vi "KB-DealWith All Picture.vi"(0 "ImageArray":T1[](array[typedef]), 5 "Param List CCD":string[][](array[string])=[[";1650.000;1055.000;162.000;324.000;0.000;0.000;0;1;3;3;15.000;4;0;1;0;0;1;65280;255;16776960;16711680;", ";1645.000;1058.000;62.000;156.000;0.000;0.000;0;1;13;13;52.000;4;0;1;0;0;1;65280;255;16776960;16711680;", "Null", "Null", "Null", "Null", "Null", "Null", "Null", "Null"], [";1666.000;992.000;164.000;329.000;0.000;0.000;0;1;3;3;12.000;4;0;1;0;0;1;65280;255;16776960;16711680;", ";1644.000;989.000;75.000;150.000;0.000;0.000;0;2;13;13;52.000;4;0;1;0;0;1;65280;255;16776960;16711680;", "Null", "Null", "Null", "Null", "Null", "Null", "Null", "Null"], [";1641.000;1097.000;175.000;301.000;0.000;0.000;0;1;3;3;12.000;4;0;1;0;0;1;65280;255;16776960;16711680;", ";1637.000;1088.000;74.000;149.000;0.000;0.000;0;2;13;13;52.000;4;0;1;0;0;1;65280;255;16776960;16711680;", "Null", "Null", "Null", "Null", "Null", "Null", "Null", "Null"], [";1645.000;1085.000;198.000;330.000;0.000;0.000;0;1;3;3;12.000;4;0;1;0;0;1;65280;255;16776960;16711680;", ";1649.000;1092.000;69.000;146.000;0.000;0.000;0;2;13;13;52.000;4;0;1;0;0;1;65280;255;16776960;16711680;", "Null", "Null", "Null", "Null", "Null", "Null", "Null", "Null"], [";1646.000;1097.000;198.000;323.000;0.000;0.000;0;1;3;3;12.000;4;0;1;0;0;1;65280;255;16776960;16711680;", ";1647.000;1093.000;74.000;149.000;0.000;0.000;0;2;19;13;52.000;4;0;1;0;0;1;65280;255;16776960;16711680;", "Null", "Null", "Null", "Null", "Null", "Null", "Null", "Null"], [";1650.000;1035.000;192.000;317.000;0.000;0.000;0;1;3;3;12.000;4;0;1;0;0;1;65280;255;16776960;16711680;", ";1669.000;1059.000;33.000;161.000;0.000;0.000;0;2;19;13;52.000;4;0;1;0;0;1;65280;255;16776960;16711680;", "Null", "Null", "Null", "Null", "Null", "Null", "Null", "Null"], [";1549.000;1024.000;204.000;306.000;0.000;0.000;0;1;3;3;12.000;4;0;1;0;0;1;65280;255;16776960;16711680;", ";1546.000;1027.000;72.000;144.000;0.000;0.000;0;2;19;13;52.000;4;0;1;0;0;1;65280;255;16776960;16711680;", "Null", "Null", "Null", "Null", "Null", "Null", "Null", "Null"], [";1552.000;926.000;174.000;303.000;0.000;0.000;0;1;19;13;52.000;4;0;1;0;0;1;65280;255;16776960;16711680;", ";1553.000;934.000;72.000;145.000;0.000;0.000;0;2;19;13;52.000;4;0;1;0;0;1;65280;255;16776960;16711680;", "Null", "Null", "Null", "Null", "Null", "Null", "Null", "Null"], [";1546.000;954.000;166.000;315.000;0.000;0.000;0;1;3;3;12.000;4;0;1;0;0;1;65280;255;16776960;16711680;", ";1547.000;950.000;73.000;147.000;0.000;0.000;0;2;19;13;52.000;4;0;1;0;0;1;65280;255;16776960;16711680;", "Null", "Null", "Null", "Null", "Null", "Null", "Null", "Null"], [";1543.000;971.000;184.000;314.000;0.000;0.000;0;1;3;3;12.000;4;0;1;0;0;1;65280;255;16776960;16711680;", ";1547.000;972.000;76.000;152.000;0.000;0.000;0;2;19;13;52.000;4;0;1;0;0;1;65280;255;16776960;16711680;", "Null", "Null", "Null", "Null", "Null", "Null", "Null", "Null"], [";1552.000;1013.000;185.000;317.000;0.000;0.000;0;1;3;3;12.000;4;0;1;0;0;1;65280;255;16776960;16711680;", ";1549.000;1013.000;72.000;145.000;0.000;0.000;0;2;19;13;52.000;4;0;1;0;0;1;65280;255;16776960;16711680;", "Null", "Null", "Null", "Null", "Null", "Null", "Null", "Null"], [";1560.000;910.000;181.000;316.000;0.000;0.000;0;1;3;3;12.000;4;0;1;0;0;1;65280;255;16776960;16711680;", ";1562.000;918.000;70.000;140.000;0.000;0.000;0;1;19;13;52.000;4;0;1;0;0;1;65280;255;16776960;16711680;", "Null", "Null", "Null", "Null", "Null", "Null", "Null", "Null"], [";1330.000;923.000;139.000;279.000;0.000;0.000;0;2;21;13;15.000;4;0;1;0;0;1;65280;255;16776960;16711680;", ";1328.000;918.000;70.000;141.000;0.000;0.000;0;2;21;13;45.000;4;0;1;0;0;1;65280;255;16776960;16711680;", "Null", "Null", "Null", "Null", "Null", "Null", "Null", "Null"], [";1370.000;1170.000;162.000;278.000;0.000;0.000;0;2;21;13;15.000;4;0;1;0;0;1;65280;255;16776960;16711680;", ";1367.000;1164.000;71.000;143.000;0.000;0.000;0;2;19;13;15.000;4;0;1;0;0;1;65280;255;16776960;16711680;", "Null", "Null", "Null", "Null", "Null", "Null", "Null", "Null"], [";1660.000;1110.000;150.000;301.000;0.000;0.000;0;2;21;13;15.000;4;0;1;0;0;1;65280;255;16776960;16711680;", ";1662.000;1114.000;78.000;156.000;0.000;0.000;0;2;21;13;25.000;4;0;1;0;0;1;65280;255;16776960;16711680;", "Null", "Null", "Null", "Null", "Null", "Null", "Null", "Null"], [";1611.000;1132.000;156.000;273.000;0.000;0.000;0;2;21;13;45.000;4;0;1;0;0;1;65280;255;16776960;16711680;", ";1613.000;1132.000;72.000;145.000;0.000;0.000;0;2;21;13;15.000;4;0;1;0;0;1;65280;255;16776960;16711680;", "Null", "Null", "Null", "Null", "Null", "Null", "Null", "Null"], [";1591.000;1169.000;165.000;294.000;0.000;0.000;0;1;13;13;15.000;4;0;1;0;0;1;65280;255;16776960;16711680;", ";1625.000;1187.000;75.000;150.000;0.000;0.000;0;2;13;13;55.000;4;0;1;0;0;1;65280;255;16776960;16711680;", "Null", "Null", "Null", "Null", "Null", "Null", "Null", "Null"], [";1586.000;1193.000;179.000;359.000;0.000;0.000;0;1;13;13;35.000;4;0;1;0;0;1;65280;255;16776960;16711680;", ";1614.000;1212.000;75.000;150.000;0.000;0.000;0;2;13;13;55.000;4;0;1;0;0;1;65280;255;16776960;16711680;", "Null", "Null", "Null", "Null", "Null", "Null", "Null", "Null"], [";1676.000;1155.000;175.000;350.000;0.000;0.000;0;1;13;13;55.000;4;0;1;0;0;1;65280;255;16776960;16711680;", ";1670.000;1157.000;70.000;141.000;0.000;0.000;0;2;13;13;55.000;4;0;1;0;0;1;65280;255;16776960;16711680;", "Null", "Null", "Null", "Null", "Null", "Null", "Null", "Null"], [";1620.000;1151.000;188.000;377.000;0.000;0.000;0;1;13;13;55.000;4;0;1;0;0;1;65280;255;16776960;16711680;", ";1613.000;1143.000;81.000;150.000;0.000;0.000;0;2;13;13;55.000;4;0;1;0;0;1;65280;255;16776960;16711680;", "Null", "Null", "Null", "Null", "Null", "Null", "Null", "Null"], [";1592.000;1152.000;179.000;359.000;0.000;0.000;0;1;13;13;55.000;4;0;1;0;0;1;65280;255;16776960;16711680;", ";1577.000;1142.000;75.000;151.000;0.000;0.000;0;2;13;13;55.000;4;0;1;0;0;1;65280;255;16776960;16711680;", "Null", "Null", "Null", "Null", "Null", "Null", "Null", "Null"], [";1284.000;1016.000;459.000;919.000;0.000;0.000;0;1;13;13;15.000;4;0;1;0;0;1;65280;255;16776960;16711680;", ";1286.000;1055.000;239.000;466.000;0.000;0.000;0;2;13;13;55.000;4;0;1;0;0;1;65280;255;16776960;16711680;", "Null", "Null", "Null", "Null", "Null", "Null", "Null", "Null"], [";1600.000;1172.000;534.000;991.000;0.000;0.000;0;1;13;13;15.000;4;0;1;0;0;1;65280;255;16776960;16711680;", ";1604.000;1188.000;203.000;406.000;0.000;0.000;0;2;15;13;43.000;4;0;1;0;0;1;65280;255;16776960;16711680;", "Null", "Null", "Null", "Null", "Null", "Null", "Null", "Null"], [";1836.000;828.000;597.000;1195.000;0.000;0.000;0;1;15;13;13.000;4;0;1;0;0;1;65280;255;16776960;16711680;", ";1840.000;824.000;216.000;432.000;0.000;0.000;0;2;5;13;43.000;4;0;1;0;0;1;65280;255;16776960;16711680;", "Null", "Null", "Null", "Null", "Null", "Null", "Null", "Null"], [";1583.000;947.000;487.000;975.000;0.000;0.000;0;1;13;13;13.000;4;0;1;0;0;1;65280;255;16776960;16711680;", ";1583.000;941.000;211.000;397.000;0.000;0.000;0;2;5;13;43.000;4;0;1;0;0;1;65280;255;16776960;16711680;", "Null", "Null", "Null", "Null", "Null", "Null", "Null", "Null"], [";1841.000;926.000;497.000;995.000;0.000;0.000;0;1;13;13;13.000;4;0;1;0;0;1;65280;255;16776960;16711680;", ";1820.000;924.000;209.000;418.000;0.000;0.000;0;2;13;13;13.000;4;0;1;0;0;1;65280;255;16776960;16711680;", "Null", "Null", "Null", "Null", "Null", "Null", "Null", "Null"], [";1728.000;864.000;582.000;1165.000;0.000;0.000;0;1;13;13;13.000;4;0;1;0;0;1;65280;255;16776960;16711680;", ";1720.000;888.000;203.000;406.000;0.000;0.000;0;2;13;13;13.000;4;0;1;0;0;1;65280;255;16776960;16711680;", "Null", "Null", "Null", "Null", "Null", "Null", "Null", "Null"], [";1508.000;1012.000;497.000;878.000;0.000;0.000;0;1;13;13;13.000;4;0;1;0;0;1;65280;255;16776960;16711680;", ";1520.000;1008.000;206.000;413.000;0.000;0.000;0;2;13;13;13.000;4;0;1;0;0;1;65280;255;16776960;16711680;", "Null", "Null", "Null", "Null", "Null", "Null", "Null", "Null"], [";2110.000;860.000;450.000;901.000;0.000;0.000;0;1;13;13;13.000;4;0;1;0;0;1;65280;255;16776960;16711680;", ";2105.000;860.000;205.000;410.000;0.000;0.000;0;2;15;13;13.000;4;0;1;0;0;1;65280;255;16776960;16711680;", "Null", "Null", "Null", "Null", "Null", "Null", "Null", "Null"], [";1900.000;1200.000;491.000;983.000;0.000;0.000;0;1;15;13;13.000;4;0;1;0;0;1;65280;255;16776960;16711680;", ";1877.000;1223.000;205.000;411.000;0.000;0.000;0;2;19;13;55.000;4;0;1;0;0;1;65280;255;16776960;16711680;", "Null", "Null", "Null", "Null", "Null", "Null", "Null", "Null"], [";2850.000;740.000;530.000;933.000;0.000;0.000;0;1;13;13;15.000;4;0;1;0;0;1;65280;255;16776960;16711680;", ";2849.000;737.000;215.000;404.000;0.000;0.000;0;2;13;13;15.000;4;0;1;0;0;1;65280;255;16776960;16711680;", "Null", "Null", "Null", "Null", "Null", "Null", "Null", "Null"], ["Null", "Null", "Null", "Null", "Null", "Null", "Null", "Null", "Null", "Null"], ["Null", "Null", "Null", "Null", "Null", "Null", "Null", "Null", "Null", "Null"]], 7 "Radio Array":string[](array[string])=["0.0079533404029692", "0.0065116279069767"], 9 "平面":i32=3000, 11 "侧面":i32=43000) -> (4 "Left Data":string[][](array[string]))   [LabVIEW 2015]
uses:
  <vilib>/vision/Image Controls.llb/IMAQ Image.ctl
panel:
  out "x/y":dbl
  out "毫秒计时值":u32
  out "路径":path
  out "数值":i32
  out "Item31":string[](array[string])
  out "Item30":string[](array[string])
  out "Item29":string[](array[string])
  out "Item28":string[](array[string])
  out "Item27":string[](array[string])
  out "Item26":string[](array[string])
  out "Item25":string[](array[string])
  out "Item24":string[](array[string])
  out "Item23":string[](array[string])
  out "Item22":string[](array[string])
  out "Item21":string[](array[string])
  out "Item20":string[](array[string])
  out "Item19":string[](array[string])
  out "Item18":string[](array[string])
  out "Item17":string[](array[string])
  out "Item16":string[](array[string])
  out "Item15":string[](array[string])
  out "Item14":string[](array[string])
  out "Item13":string[](array[string])
  out "Item12":string[](array[string])
  out "Item11":string[](array[string])
  out "Item10":string[](array[string])
  out "Item9":string[](array[string])
  out "Item8":string[](array[string])
  out "Item7":string[](array[string])
  out "Item6":string[](array[string])
  out "Item5":string[](array[string])
  out "Item4":string[](array[string])
  out "Item3":string[](array[string])
  out "Item2":string[](array[string])
  out "Item1":string[](array[string])
  out "CCD 2":string
  out "CCD 1":string
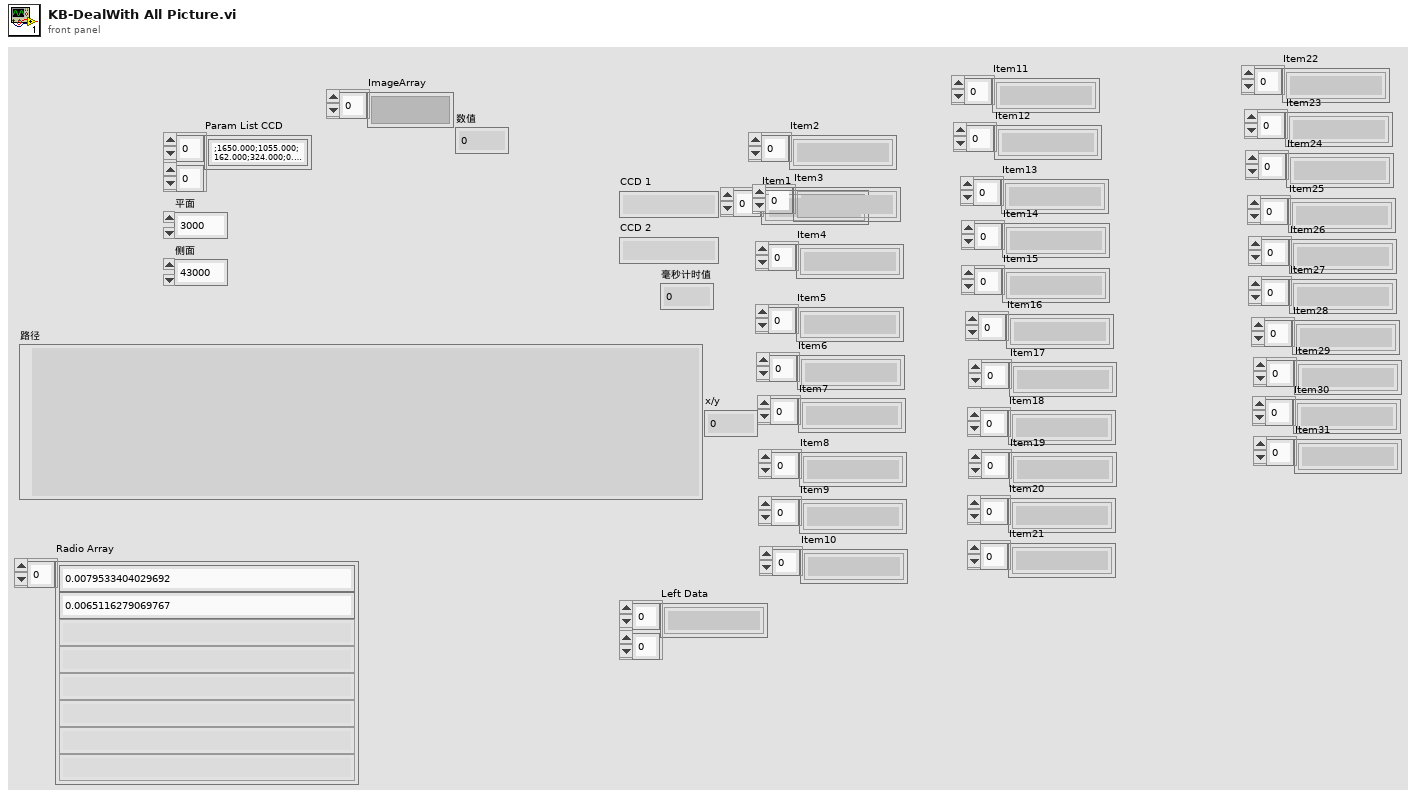
[diagram p1: front panel]
types:
  T1 = typedef "IMAQ Image.ctl" = refnum<image>
  T2 = typedef "Image Type" = u32
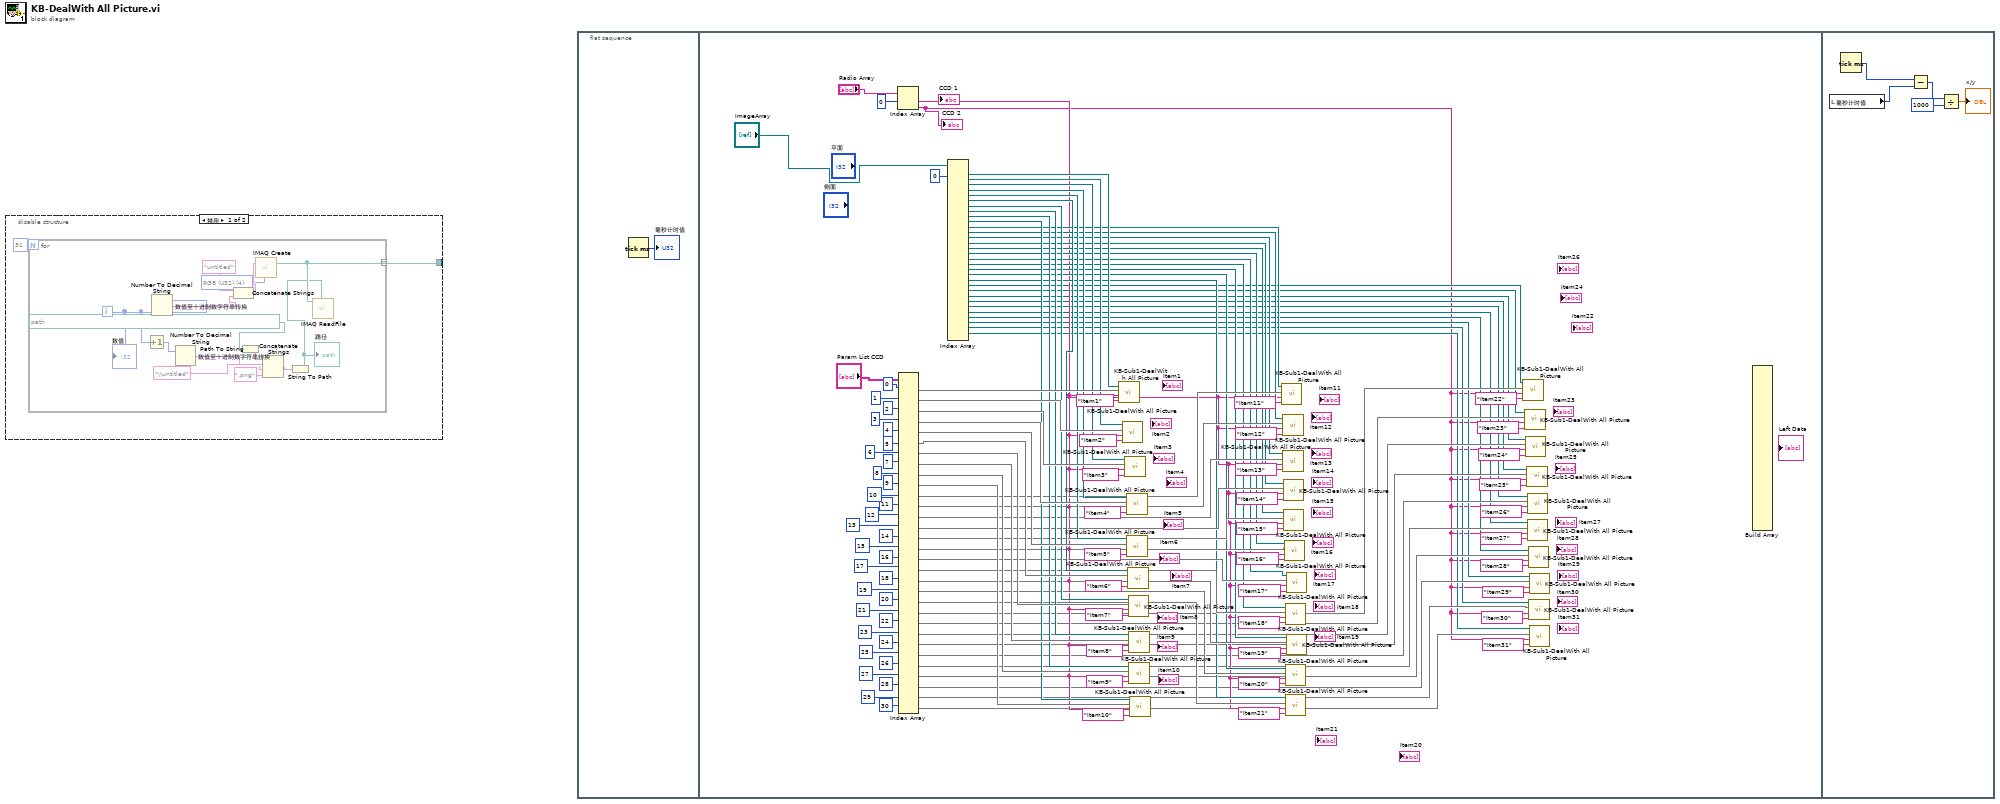
[diagram p0: block diagram]
diagram:
  n1 = disable-structure shown="禁用" {
    disable-tunnel: [w1 _] -> _
    frame Disabled {
      n2 = for {
        N: 31 -> [_]
        tunnel: [w13] -> w1 mode=indexing
        i -> [w5]
        w14 = T2 4 items=["Grayscale (U8)", "Grayscale (I16)", "Grayscale (SGL)", "Complex (CSG)", "RGB (U32)", "HSL (U32)", "RGB (U64)", "Grayscale (U16)"] ("Image Type")
        n3 = Increment(x=w5) -> (x+1=w4:i32)
        n4 = Number To Decimal String "数值至十进制数字符串转换"(number=w5) -> (decimal integer string=w9:string)  [unwired: 1 in]
        n5 = Number To Decimal String "数值至十进制数字符串转换"(number=w4) -> (decimal integer string=w3:string)  [unwired: 1 in]
        n6 = Concatenate Strings("untitled" ("Image Name"), w9) -> (w15:string)
        n7 = Path To String(path=path "C:/Users/Administrator.PC-20160727FSNO/Desktop/新建文件夹" ("File Path")) -> (string=w11:string)
        n8 = call "IMAQ Create"("Image Name"=w15, "Image Type"=w14) -> ("New Image"=w13:T1)  [unwired: 3 in, 1 out]
        n9 = Concatenate Strings(w11, "\\untitled" ("字符串"), w3, ".png" ("字符串")) -> (w7:string)
        n10 = String To Path(string=w7) -> (path=w6:path)
        "路径" <- w6
        n11 = call "IMAQ ReadFile"("File Path"=w6, "Image"=w13) -> ()  [unwired: 5 in, 5 out]
        "数值" <- w5
      }
    }
    frame Enabled {
    }
  }
  n12 = flat-sequence {
    frame #0 {
      n13 = Tick Count (ms)() -> (millisecond timer value=→"毫秒计时值":u32)
    }
    frame #1 {
      n14 = Index Array(array="Radio Array", index #1=0 ("索引")) -> (element #1=w51:string, element #2=w20:string)  [unwired: 1 in]
      "CCD 1" <- w51
      "CCD 2" <- w20
      n15 = Index Array(array="Param List CCD", index (row) #1=0 ("索引 (行)"), index (row) #2=1 ("索引 (行)"), index (row) #3=2 ("索引 (行)"), index (row) #4=3 ("索引 (行)"), index (row) #5=4 ("索引 (行)"), index (row) #6=5 ("索引 (行)"), index (row) #7=6 ("索引 (行)"), index (row) #8=7 ("索引 (行)"), index (row) #9=8 ("索引 (行)"), index (row) #10=9 ("索引 (行)"), index (row) #11=10 ("索引 (行)"), index (row) #12=11 ("索引 (行)"), index (row) #13=12 ("索引 (行)"), index (row) #14=13 ("索引 (行)"), index (row) #15=14 ("索引 (行)"), index (row) #16=15 ("索引 (行)"), index (row) #17=16 ("索引 (行)"), index (row) #18=17 ("索引 (行)"), index (row) #19=18 ("索引 (行)"), index (row) #20=19 ("索引 (行)"), index (row) #21=20 ("索引 (行)"), index (row) #22=21 ("索引 (行)"), index (row) #23=22 ("索引 (行)"), index (row) #24=23 ("索引 (行)"), index (row) #25=24 ("索引 (行)"), index (row) #26=25 ("索引 (行)"), index (row) #27=26 ("索引 (行)"), index (row) #28=27 ("索引 (行)"), index (row) #29=28 ("索引 (行)"), index (row) #30=29 ("索引 (行)"), index (row) #31=30 ("索引 (行)")) -> (element #1=w144:string[], element #2=w138:string[], element #3=w135:string[], element #4=w103:string[], element #5=w100:string[], element #6=w97:string[], element #7=w94:string[], element #8=w91:string[], element #9=w88:string[], element #10=w85:string[], element #11=w82:string[], element #12=w79:string[], element #13=w76:string[], element #14=w73:string[], element #15=w71:string[], element #16=w69:string[], element #17=w64:string[], element #18=w61:string[], element #19=w58:string[], element #20=w55:string[], element #21=w52:string[], element #22=w48:string[], element #23=w45:string[], element #24=w42:string[], element #25=w39:string[], element #26=w36:string[], element #27=w33:string[], element #28=w30:string[], element #29=w28:string[], element #30=w24:string[], element #31=w21:string[])  [unwired: 31 in]
      n16 = Index Array(array="ImageArray", index #1=0 ("索引")) -> (element #1=w143:T1, element #2=w139:T1, element #3=w134:T1, element #4=w104:T1, element #5=w101:T1, element #6=w98:T1, element #7=w95:T1, element #8=w92:T1, element #9=w89:T1, element #10=w86:T1, element #11=w83:T1, element #12=w80:T1, element #13=w77:T1, element #14=w74:T1, element #15=w72:T1, element #16=w67:T1, element #17=w65:T1, element #18=w62:T1, element #19=w59:T1, element #20=w56:T1, element #21=w53:T1, element #22=w49:T1, element #23=w46:T1, element #24=w43:T1, element #25=w40:T1, element #26=w37:T1, element #27=w34:T1, element #28=w31:T1, element #29=w29:T1, element #30=w25:T1, element #31=w22:T1)  [unwired: 31 in, 1 out]
      n17 = call "KB-Sub1-DealWith All Picture.vi"("Row Select"="Item1", "相机分辨率"=w51, "参数"=w144, "Image  In"=w143) -> ()  [unwired: 4 in, 4 out]
      n18 = call "KB-Sub1-DealWith All Picture.vi"("Row Select"="Item2", "相机分辨率"=w51, "参数"=w138, "Image  In"=w139) -> ()  [unwired: 4 in, 4 out]
      n19 = call "KB-Sub1-DealWith All Picture.vi"("Row Select"="Item3", "相机分辨率"=w51, "参数"=w135, "Image  In"=w134) -> ()  [unwired: 4 in, 4 out]
      n20 = call "KB-Sub1-DealWith All Picture.vi"("Row Select"="Item4", "相机分辨率"=w51, "参数"=w103, "Image  In"=w104) -> ()  [unwired: 4 in, 4 out]
      n21 = call "KB-Sub1-DealWith All Picture.vi"("Row Select"="Item5", "相机分辨率"=w51, "参数"=w100, "Image  In"=w101) -> ()  [unwired: 4 in, 4 out]
      n22 = call "KB-Sub1-DealWith All Picture.vi"("Row Select"="Item6", "相机分辨率"=w51, "参数"=w97, "Image  In"=w98) -> ()  [unwired: 4 in, 4 out]
      n23 = call "KB-Sub1-DealWith All Picture.vi"("Row Select"="Item7", "相机分辨率"=w51, "参数"=w94, "Image  In"=w95) -> ()  [unwired: 4 in, 4 out]
      n24 = call "KB-Sub1-DealWith All Picture.vi"("Row Select"="Item8", "相机分辨率"=w51, "参数"=w91, "Image  In"=w92) -> ()  [unwired: 4 in, 4 out]
      n25 = call "KB-Sub1-DealWith All Picture.vi"("Row Select"="Item9", "相机分辨率"=w51, "参数"=w88, "Image  In"=w89) -> ()  [unwired: 4 in, 4 out]
      n26 = call "KB-Sub1-DealWith All Picture.vi"("Row Select"="Item10", "相机分辨率"=w51, "参数"=w85, "Image  In"=w86) -> ()  [unwired: 4 in, 4 out]
      n27 = call "KB-Sub1-DealWith All Picture.vi"("Row Select"="Item11", "相机分辨率"=w51, "参数"=w82, "Image  In"=w83) -> ()  [unwired: 4 in, 4 out]
      n28 = call "KB-Sub1-DealWith All Picture.vi"("Row Select"="Item12", "相机分辨率"=w51, "参数"=w79, "Image  In"=w80) -> ()  [unwired: 4 in, 4 out]
      n29 = call "KB-Sub1-DealWith All Picture.vi"("Row Select"="Item13", "相机分辨率"=w51, "参数"=w76, "Image  In"=w77) -> ()  [unwired: 4 in, 4 out]
      n30 = call "KB-Sub1-DealWith All Picture.vi"("Row Select"="Item14", "相机分辨率"=w51, "参数"=w73, "Image  In"=w74) -> ()  [unwired: 4 in, 4 out]
      n31 = call "KB-Sub1-DealWith All Picture.vi"("Row Select"="Item15", "相机分辨率"=w51, "参数"=w71, "Image  In"=w72) -> ()  [unwired: 4 in, 4 out]
      n32 = call "KB-Sub1-DealWith All Picture.vi"("Row Select"="Item16", "相机分辨率"=w51, "参数"=w69, "Image  In"=w67) -> ()  [unwired: 4 in, 4 out]
      n33 = call "KB-Sub1-DealWith All Picture.vi"("Row Select"="Item18", "相机分辨率"=w51, "参数"=w61, "Image  In"=w62) -> ()  [unwired: 4 in, 4 out]
      n34 = call "KB-Sub1-DealWith All Picture.vi"("Row Select"="Item20", "相机分辨率"=w51, "参数"=w55, "Image  In"=w56) -> ()  [unwired: 4 in, 4 out]
      n35 = call "KB-Sub1-DealWith All Picture.vi"("Row Select"="Item21", "相机分辨率"=w51, "参数"=w52, "Image  In"=w53) -> ()  [unwired: 4 in, 4 out]
      n36 = call "KB-Sub1-DealWith All Picture.vi"("Row Select"="Item17", "相机分辨率"=w51, "参数"=w64, "Image  In"=w65) -> ()  [unwired: 4 in, 4 out]
      n37 = call "KB-Sub1-DealWith All Picture.vi"("Row Select"="Item19", "相机分辨率"=w51, "参数"=w58, "Image  In"=w59) -> ()  [unwired: 4 in, 4 out]
      n38 = call "KB-Sub1-DealWith All Picture.vi"("Row Select"="Item22", "相机分辨率"=w20, "参数"=w48, "Image  In"=w49) -> ()  [unwired: 4 in, 4 out]
      n39 = call "KB-Sub1-DealWith All Picture.vi"("Row Select"="Item23", "相机分辨率"=w20, "参数"=w45, "Image  In"=w46) -> ()  [unwired: 4 in, 4 out]
      n40 = call "KB-Sub1-DealWith All Picture.vi"("Row Select"="Item24", "相机分辨率"=w20, "参数"=w42, "Image  In"=w43) -> ()  [unwired: 4 in, 4 out]
      n41 = call "KB-Sub1-DealWith All Picture.vi"("Row Select"="Item25", "相机分辨率"=w20, "参数"=w39, "Image  In"=w40) -> ()  [unwired: 4 in, 4 out]
      n42 = call "KB-Sub1-DealWith All Picture.vi"("Row Select"="Item26", "相机分辨率"=w20, "参数"=w36, "Image  In"=w37) -> ()  [unwired: 4 in, 4 out]
      n43 = call "KB-Sub1-DealWith All Picture.vi"("Row Select"="Item27", "相机分辨率"=w20, "参数"=w33, "Image  In"=w34) -> ()  [unwired: 4 in, 4 out]
      n44 = call "KB-Sub1-DealWith All Picture.vi"("Row Select"="Item28", "相机分辨率"=w20, "参数"=w30, "Image  In"=w31) -> ()  [unwired: 4 in, 4 out]
      n45 = call "KB-Sub1-DealWith All Picture.vi"("Row Select"="Item30", "相机分辨率"=w20, "参数"=w24, "Image  In"=w25) -> ()  [unwired: 4 in, 4 out]
      n46 = call "KB-Sub1-DealWith All Picture.vi"("Row Select"="Item29", "相机分辨率"=w20, "参数"=w28, "Image  In"=w29) -> ()  [unwired: 4 in, 4 out]
      n47 = call "KB-Sub1-DealWith All Picture.vi"("Row Select"="Item31", "相机分辨率"=w20, "参数"=w21, "Image  In"=w22) -> ()  [unwired: 4 in, 4 out]
      n48 = Build Array() -> ()  [unwired: 31 in, 1 out]
    }
    frame #2 {
      n49 = local read "毫秒计时值"() -> (w152:u32)
      n50 = Tick Count (ms)() -> (millisecond timer value=w153:u32)
      n51 = Subtract(x=w153, y=w152) -> (x-y=w151:u32)
      n52 = Divide(x=w151, y=u32 1000) -> (x/y=→"x/y":dbl)
    }
  }
